vi "Get as Timestamp.vi"(8 "error in (no error)":errorcluster, 10 "Name Array":string[](array[string]), 11 "JSON Value in":refnum<class "JSON Value.lvclass">) -> (0 "error out":errorcluster, 2 "Time Stamp":timestamp, 3 "JSON Value out":refnum<class "JSON Value.lvclass">)   [LabVIEW 2011, in "JSON Scalar.lvclass"]
doc: "Converts a <b>JSON Value</b> into a <b>Time Stamp</b>.\nUses different timestamp formatters to retrieve a timestamp.\n\nCopyright 2012 James David Powell, Shaun Rumbell and Ton Plomp\nMore information on http://lavag.org/topic/16217-cr-json-labview"
uses:
  JSON Scalar.lvclass
  JSON Value/JSON Value.lvclass
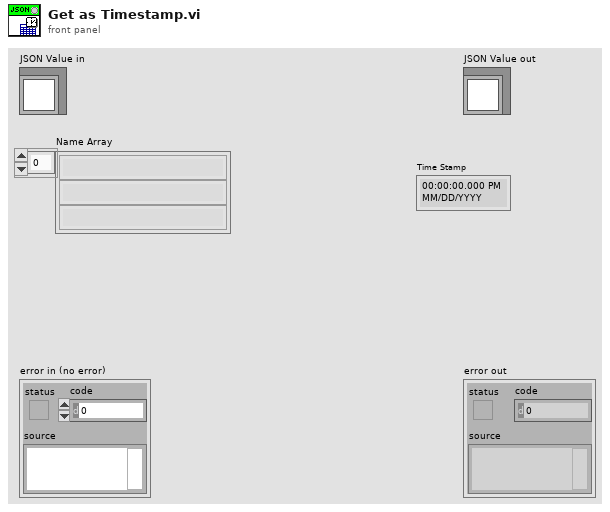
[diagram p1: front panel]
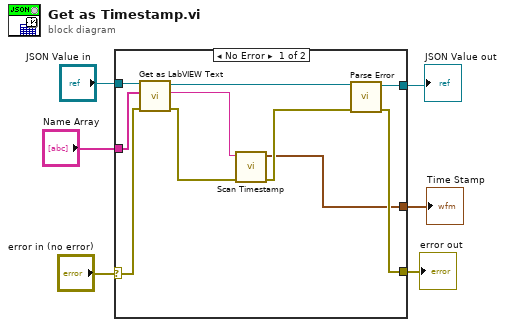
[diagram p0: block diagram]
diagram:
  n1 = case shown="No Error" "error in (no error)" {
    selector: "error in (no error)" -> [w12 w18]
    tunnel: [w8 _] -> w6
    tunnel: "JSON Value in" -> [w16 w17]
    tunnel: [w14 w17] -> w4
    tunnel: [w13 w18] -> w3
    tunnel: "Name Array" -> [w7 _]
    frame No Error {
      n2 = call-dynamic "Get as LabVIEW Text.vi"("error in (no error)"=w12, "Name Array"=w7, "JSON Value In"=w16) -> ("error out"=w10:errorcluster, "LabVIEW Text"=w11:string, "JSON Value Out"=w15:refnum<class "JSON Value.lvclass">)  [unwired: 6 in]
      n3 = call "Scan Timestamp.vi"("error in (no error)"=w10, "String"=w11) -> ("error out"=w9:errorcluster, "Timestamp"=w8:timestamp)  [unwired: 8 in]
      n4 = call-dynamic "Parse Error.vi"("error in (no error)"=w9, "JSON Value in"=w15) -> ("error out"=w13:errorcluster, "JSON Value out"=w14:refnum<class "JSON Value.lvclass">)  [unwired: 8 in]
    }
    frame Error {
    }
  }
  "error out" <- w3
  "JSON Value out" <- w4
  "Time Stamp" <- w6
